vi "Autobalance Data DAO.vi"(8 "error in (no error)":errorcluster, 9 "L2 Autobalance In":T2[](array[typedef]), 10 "L1 Autobalance Iin":T2[](array[typedef]), 11 "DAO Actions":T1) -> (0 "error out":errorcluster, 1 "L2 Autobalance Out":T2[](array[typedef]), 2 "L1 Autobalance Out":T2[](array[typedef]))   [LabVIEW 2009]
uses:
  Autobalance Status Data.ctl
  Apps/Yes No Button.ctl
  Autobalance Stage.ctl
  Autobalance Data Point.ctl
  Data Access Objects/Metadata/DAO Actions.ctl
panel:
  # "Cmd"
  # "Servo"
  # "Cmd"
  # "Servo"
  # "Cmd"
  # "Servo"
  # "Cmd"
  # "Servo"
  # "Cmd"
  # "Servo"
  # "Cmd"
  # "Servo"
  # "Cmd"
  # "Servo"
  # "Cmd"
  # "Servo"
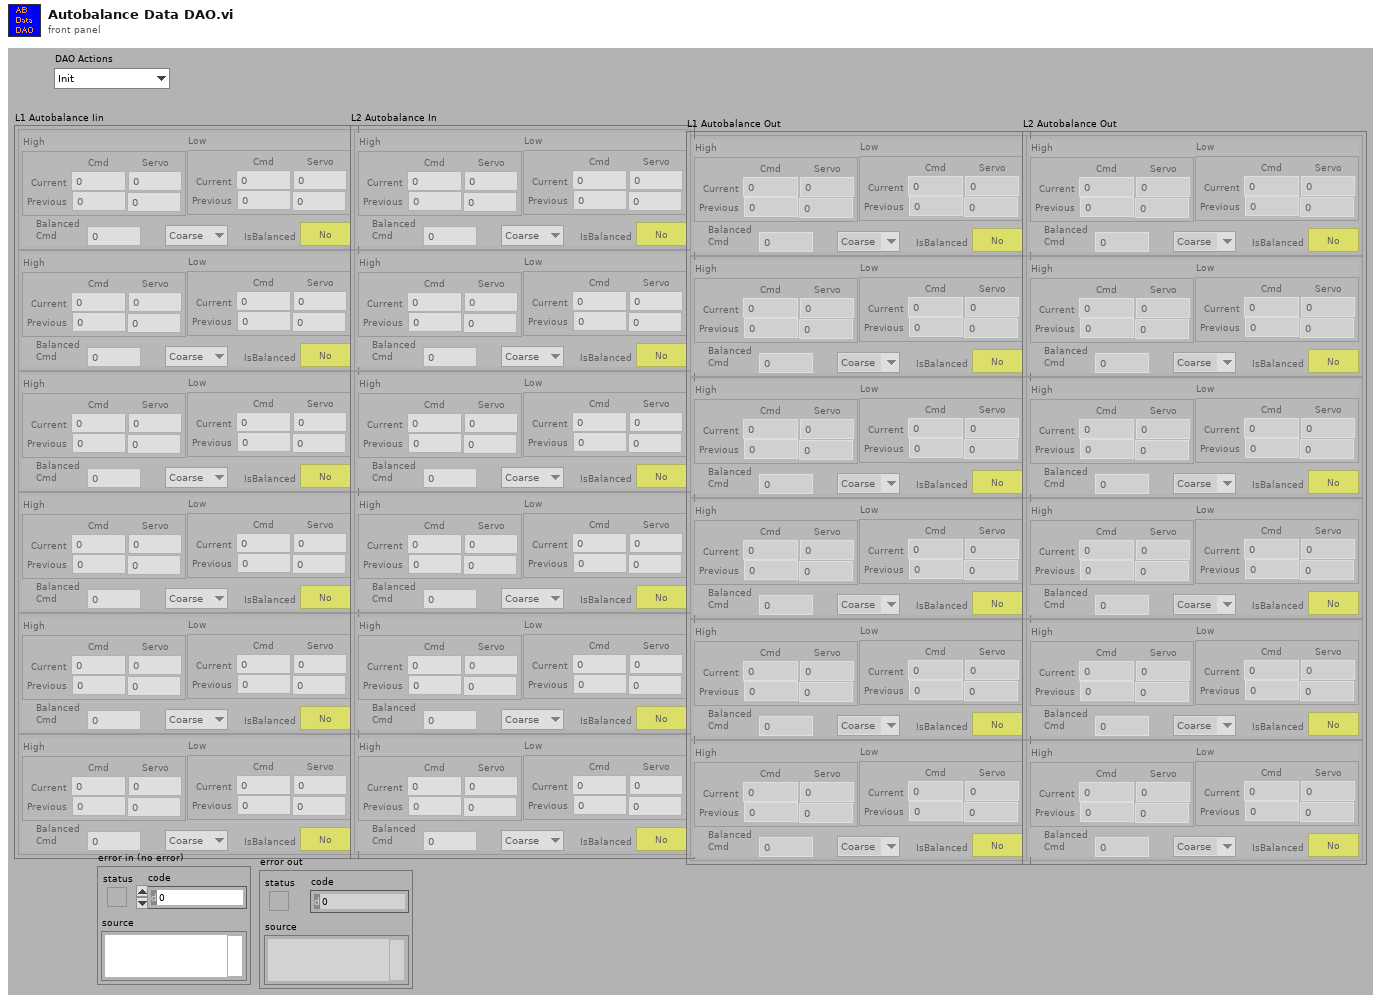
[diagram p1: front panel]
types:
  T1 = typedef "DAO Actions.ctl" = enum16{"Init", "Get", "Set"}
  T2 = typedef "Autobalance Status Data.ctl" = cluster{"IsBalanced":T3, "Autobalance Stage":T4, "High":T5, "Low":T5, "Balanced \nCmd":dbl}
  T3 = typedef "Yes No Button.ctl" = bool
  T4 = typedef "Autobalance Stage.ctl" = enum16{"Coarse", "Medium", "Fine", "Done"}
  T5 = typedef "Autobalance Data Point.ctl" = cluster{"cCmd":dbl, "cServo":dbl, "pCmd":dbl, "pServo":dbl}
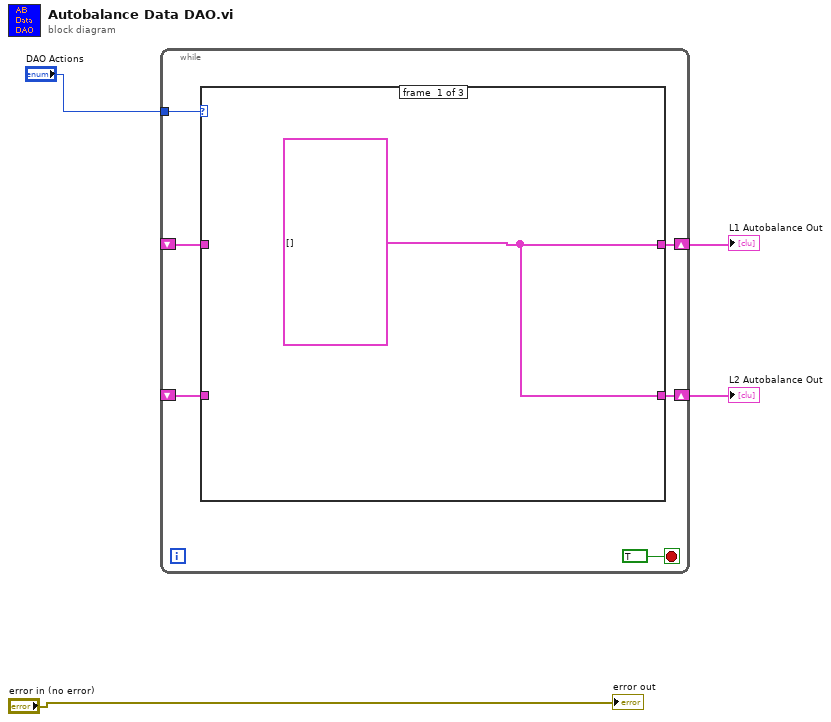
[diagram p0: block diagram]
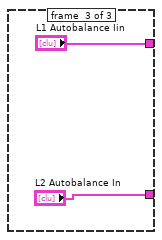
[diagram p3: hidden frame]
diagram:
  n1 = while {
    tunnel: "DAO Actions" -> [w9]
    shift-right: [w8] -> w2
    shift-left: _ -> [w6]
    shift-right: [w7] -> w1
    shift-left: _ -> [w5]
    stop <- TRUE stop-if-true
    n2 = case shown="\"Set\"" w9 {
      tunnel: [w11 w13 "L1 Autobalance Iin"] -> w8
      tunnel: [w11 w12 "L2 Autobalance In"] -> w7
      tunnel: w6 -> [_ w13 _]
      tunnel: w5 -> [_ w12 _]
      frame #0 {
        w11 = T2[] [] ("L1 Autobalance Iin")
      }
      frame #1 {
      }
      frame #2 {
      }
    }
  }
  "L1 Autobalance Out" <- w2
  "L2 Autobalance Out" <- w1
  "error out" <- "error in (no error)"
